vi "2-bit-flipflop.vi"() -> ()   [LabVIEW 2024]
uses:
  controls/4-bit-disp.ctl
  controls/7-segment-display.ctl
  controls/!4-bit-cont.ctl
panel:
  out "7-segment":T1
  out "Iteration":i32
  out "!4-bit-display":T2
  out "4-bit-display":T3
  in  "Stop Button":bool
  in  "CLK":bool
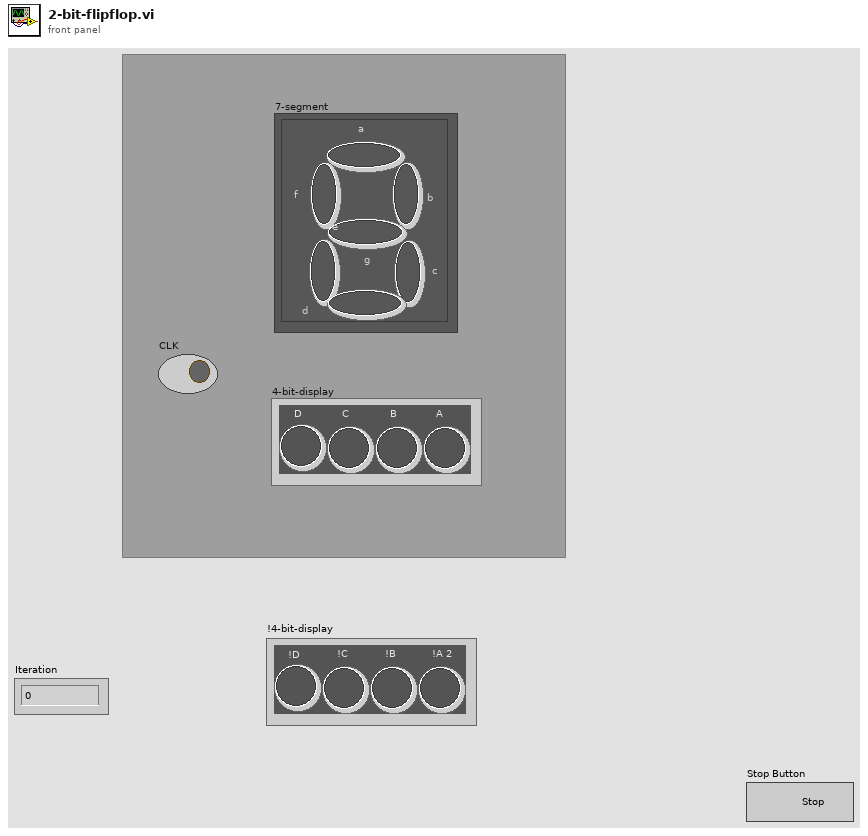
[diagram p1: front panel]
types:
  T1 = typedef "7-segment-display.ctl" = cluster{"a":bool, "b":bool, "c":bool, "d":bool, "e":bool, "f":bool, "g":bool}
  T2 = cluster{"!D":bool, "!C":bool, "!B":bool, "!A 2":bool}
  T3 = typedef "4-bit-disp.ctl" = cluster{"D":bool, "C":bool, "B":bool, "A":bool}
  T4 = typedef "!4-bit-cont.ctl" = cluster{"!D":bool, "!C":bool, "!B":bool, "!A":bool}
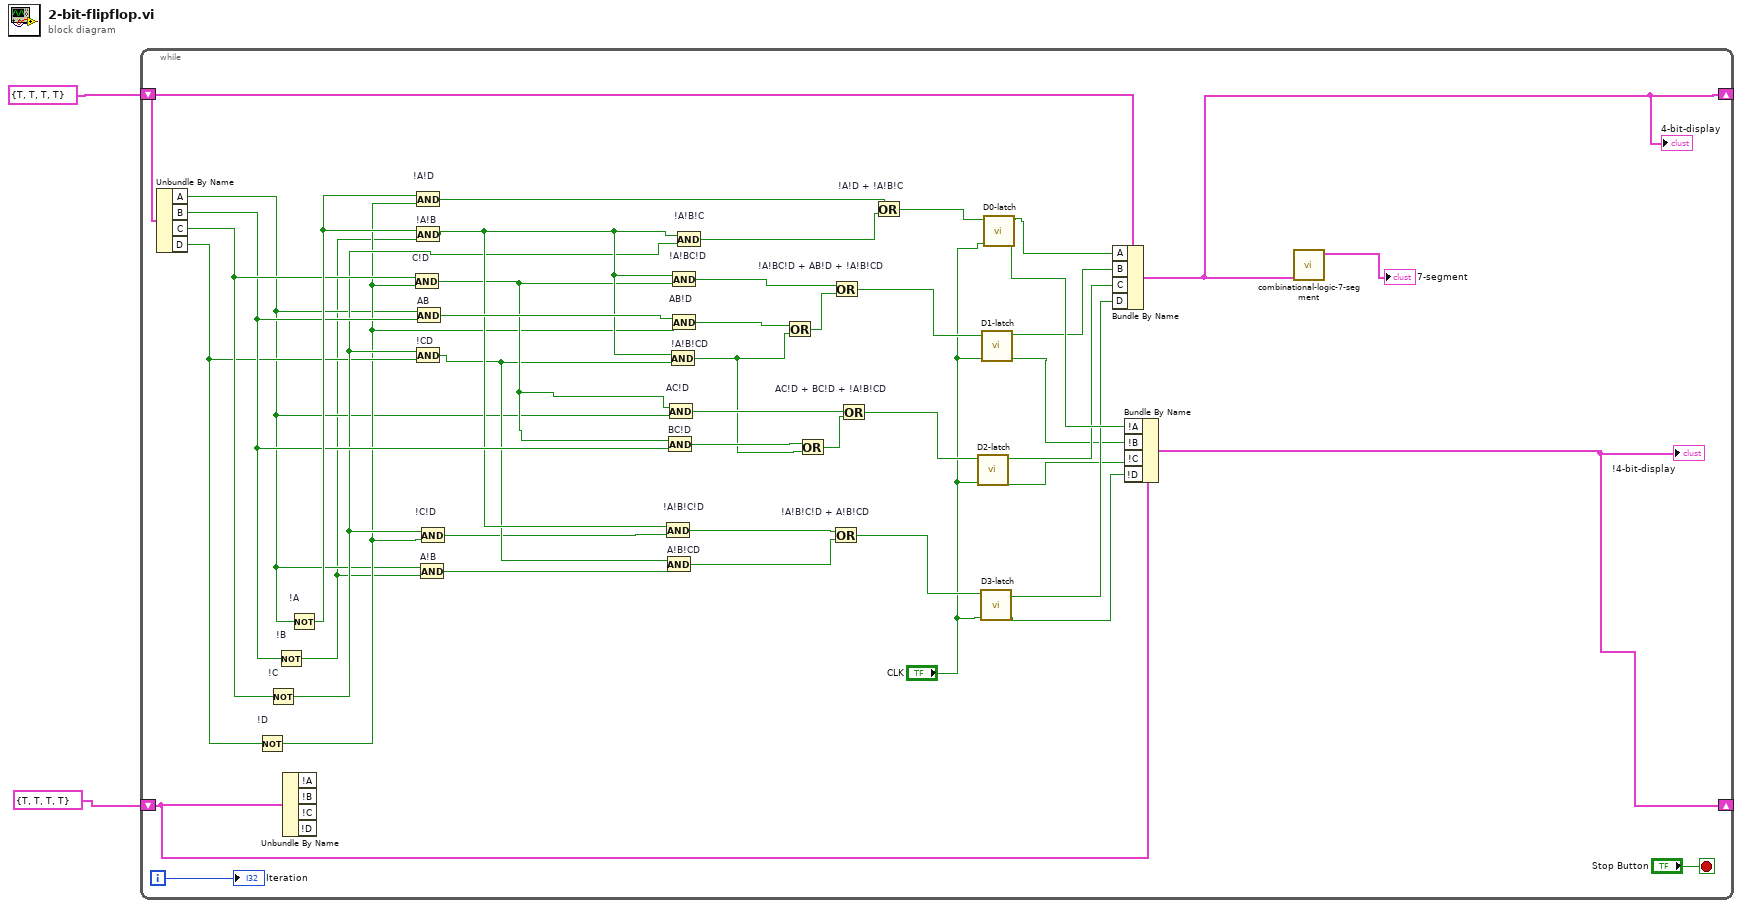
[diagram p0: block diagram]
diagram:
  n1 = while {
    shift-right: [w30] -> _
    shift-left: T3 {"D"=TRUE, "C"=TRUE, "B"=TRUE, "A"=TRUE} ("4-bit-display") -> [w46]
    shift-right: [w44] -> _
    shift-left: T4 {"!D"=TRUE, "!C"=TRUE, "!B"=TRUE, "!A"=TRUE} ("4-bit-display") -> [w45]
    i -> [w43]
    stop <- "Stop Button" stop-if-true
    n2 = Unbundle By Name(w46) -> ("A"=w4:bool, "B"=w17:bool, "C"=w21:bool, "D"=w11:bool)
    n3 = Not "!D"(x=w11) -> (.not. x?=w7:bool)
    n4 = Not "!C"(x=w21) -> (.not. x?=w12:bool)
    n5 = Not "!B"(x=w17) -> (.not. x?=w3:bool)
    n6 = Unbundle By Name(w45) -> ()  [unwired: 4 out]
    n7 = Not "!A"(x=w4) -> (.not. x?=w24:bool)
    n8 = And "C!D"(x=w21, y=w7) -> (x .and. y?=w13:bool)
    n9 = And "!A!D"(x=w24, y=w7) -> (x .and. y?=w29:bool)
    n10 = And "!A!B"(x=w24, y=w3) -> (x .and. y?=w16:bool)
    n11 = And "!CD"(x=w12, y=w11) -> (x .and. y?=w9:bool)
    n12 = And "AB"(x=w4, y=w17) -> (x .and. y?=w25:bool)
    n13 = And "A!B"(x=w4, y=w3) -> (x .and. y?=w6:bool)
    n14 = And "!C!D"(x=w12, y=w7) -> (x .and. y?=w8:bool)
    n15 = And "!A!B!C!D"(x=w16, y=w8) -> (x .and. y?=w23:bool)
    n16 = And "A!B!CD"(x=w9, y=w6) -> (x .and. y?=w5:bool)
    n17 = And "BC!D"(x=w13, y=w17) -> (x .and. y?=w18:bool)
    n18 = And "AC!D"(x=w13, y=w4) -> (x .and. y?=w19:bool)
    n19 = And "!A!B!CD"(x=w16, y=w9) -> (x .and. y?=w10:bool)
    n20 = And "!A!BC!D"(x=w16, y=w13) -> (x .and. y?=w28:bool)
    n21 = And "AB!D"(x=w25, y=w7) -> (x .and. y?=w26:bool)
    n22 = And "!A!B!C"(x=w16, y=w12) -> (x .and. y?=w22:bool)
    n23 = Or(x=w26, y=w10) -> (x .or. y?=w27:bool)
    n24 = Or(x=w18, y=w10) -> (x .or. y?=w20:bool)
    n25 = Or "!A!B!C!D + A!B!CD"(x=w23, y=w5) -> (x .or. y?=w38:bool)
    n26 = Or "!A!BC!D + AB!D + !A!B!CD"(x=w28, y=w27) -> (x .or. y?=w35:bool)
    n27 = Or "AC!D + BC!D + !A!B!CD"(x=w19, y=w20) -> (x .or. y?=w37:bool)
    n28 = Or "!A!D + !A!B!C"(x=w29, y=w22) -> (x .or. y?=w32:bool)
    n29 = call "D2-latch.vi"("CLK"="CLK", "D"=w37) -> ("'Q"=w15:bool, "Q"=w36:bool)  [unwired: 8 in]
    n30 = call "D3-latch.vi"("CLK"="CLK", "D"=w38) -> ("'Q"=w39:bool, "Q"=w40:bool)  [unwired: 8 in]
    n31 = call "D1-latch.vi"("CLK"="CLK", "D"=w35) -> ("'Q"=w34:bool, "Q"=w33:bool)  [unwired: 8 in]
    n32 = call "D0-latch.vi"("CLK"="CLK", "D"=w32) -> ("'Q"=w41:bool, "Q"=w42:bool)  [unwired: 8 in]
    n33 = Bundle By Name(cluster=w46, "A"=w42, "B"=w33, "C"=w36, "D"=w40) -> (w30:T3)
    "4-bit-display" <- w30
    n34 = Bundle By Name(cluster=w45, "!A"=w41, "!B"=w34, "!C"=w15, "!D"=w39) -> (w44:T4)
    "!4-bit-display" <- w44
    n35 = call "combinational-logic-7-segment.vi"("4-bit-reg-input"=w30) -> ("7-segment CTRL out"=→"7-segment":T1)  [unwired: 9 in, 1 out]
    "Iteration" <- w43
  }
